vi "3. MassData in Non-CSM Framework.vi"() -> ()   [LabVIEW 2017]
uses:
  addons/MassData-Parameter/Utility/Def-MassData Status Indicator(Vertical).ctl
  35609cad-7792-4b26-abfa-db0d207ea277.vi
  216db254-1a31-45ab-afe3-8c3bb1289dd0.vi
  addons/MassData-Parameter/_support/FGV-MassData(lvlibp).vi
  addons/MassData-Parameter/CSM MassData Parameter Support.lvlib
panel:
  in  "Generate":bool
  out "MassData Status Vertical":T1={"w"={287840.0, 276144.0}, "r"={287840.0, 276144.0}} {"r" scale=1.0..5000000.0 scale format="%#_6p"; "w" scale=1.0..5000000.0 scale format="%#_6p"}
  out "Waveform Graph":waveform(dbl)(graph)
  in  "stop":bool
  # "#CSM-Example overview"
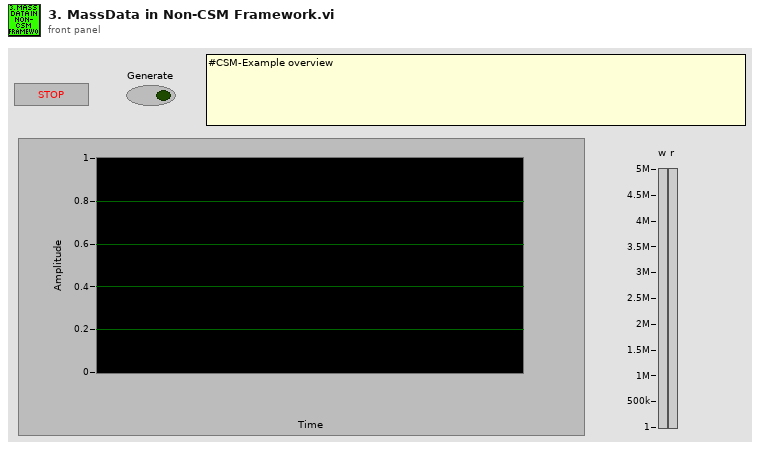
[diagram p1: front panel]
types:
  T1 = typedef "Def-MassData Status Indicator(Vertical).ctl" = cluster{"w":cluster{dbl, dbl}, "r":cluster{dbl, dbl}}
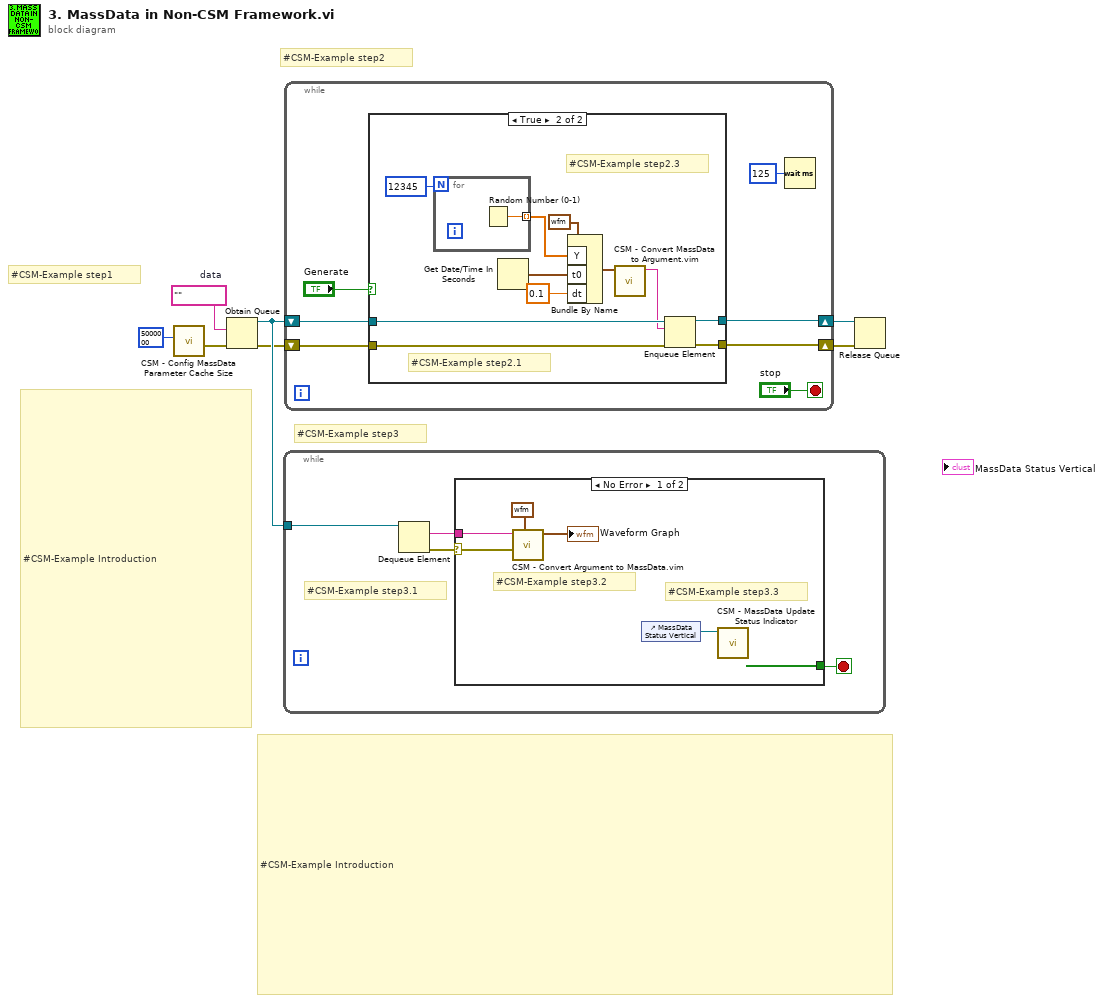
[diagram p0: block diagram]
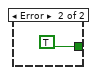
[diagram p2: hidden frame]
diagram:
  w3 = ""  # data
  # "#CSM-Example step3"
  # "#CSM-Example step2"
  # "#CSM-Example step1"
  # "#CSM-Example Introduction"
  # "#CSM-Example Introduction"
  n1 = call "CSM - Config MassData Parameter Cache Size.vi"("size(1M)"=5000000) -> ("Error out"=w1:errorcluster)  [unwired: 10 in]
  n2 = Obtain Queue(element data type=w3, error in (no error)=w1) -> (queue out=w7:refnum<queue>, error out=w6:errorcluster)  [unwired: 3 in, 1 out]
  n3 = while {
    tunnel: w7 -> [w11]
    stop <- w8 stop-if-true
    # "#CSM-Example step3.1"
    n4 = Dequeue Element(queue=w11) -> (element=w9:string, error out=w10:errorcluster)  [unwired: 2 in, 2 out]
    n5 = case shown="No Error" w10 {
      selector: w10 -> [w14 _]
      tunnel: w9 -> [w13 _]
      tunnel: [_ TRUE] -> w8
      frame No Error {
        # "#CSM-Example step3.3"
        # "#CSM-Example step3.2"
        n6 = call "CSM - Convert Argument to MassData.vim"("Type"=waveform(dbl) {"t0"=timestamp(0 s since 1904-01-01), "dt"=1.0, "Y"=[]} ("output waveform"), "error in (no error)"=w14, "MassData Argument"=w13) -> ("Data"=→"Waveform Graph":waveform(dbl))  [unwired: 5 in, 1 out]
        n7 = control-ref of="MassData Status Vertical"() -> (w16:refnum<vi>)
        n8 = call "CSM - MassData Update Status Indicator.vi"("MassData Status Indicator"=w16) -> ()  [unwired: 10 in, 1 out]
      }
      frame Error {
      }
    }
  }
  n9 = while {
    shift-right: [w20] -> w4
    shift-left: w6 -> [w21]
    shift-right: [w22] -> w5
    shift-left: w7 -> [w23]
    stop <- "stop" stop-if-true
    n10 = case shown="True" "Generate" {
      tunnel: w23 -> [w26 w37]
      tunnel: [w26 w36] -> w22
      tunnel: w21 -> [w25 w35]
      tunnel: [w25 w34] -> w20
      frame False {
      }
      frame True {
        # "#CSM-Example step2.3"
        # "#CSM-Example step2.1"
        n11 = for {
          N: 12345 -> [_]
          tunnel: [w38] -> w33 mode=indexing
          n12 = Random Number (0-1)() -> (number: 0 to 1=w38:dbl)
        }
        n13 = Get Date/Time In Seconds() -> (seconds since 1Jan1904=w32:timestamp)
        n14 = Bundle By Name(cluster=waveform(dbl) {"t0"=timestamp(0 s since 1904-01-01), "dt"=1.0, "Y"=[]} ("Waveform"), "Y"=w33, "t0"=w32, "dt"=0.1) -> (w28:waveform(dbl))
        n15 = call "CSM - Convert MassData to Argument.vim"("DBL"=w28) -> ("MassData Argument"=w27:string)  [unwired: 7 in, 1 out]
        n16 = Enqueue Element(queue=w37, element=w27, error in (no error)=w35) -> (queue out=w36:refnum<queue>, error out=w34:errorcluster)  [unwired: 1 in, 1 out]
      }
    }
    n17 = Wait (ms)(milliseconds to wait=u32 125) -> ()  [unwired: 1 out]
  }
  n18 = Release Queue(queue=w5, error in (no error)=w4) -> ()  [unwired: 1 in, 3 out]
